vi "Actor Core.vi"(8 "error in":errorcluster, 11 "RandomDataChart in":refnum<class "AutoRegPanel.lvclass">) -> (0 "error out":errorcluster, 3 "Actor out":refnum<class "Actor.lvclass">)   [LabVIEW 2015, in "TestViewables.lvlib" / "AutoRegPanel.lvclass"]
doc: "(<B>Filename</B>: Actor Framework.lvlib:Actor.lvclass:Actor Core.vi)\n\nReceives messages to the actor, reacts to them, and initiates any error handling that may shut the actor down.\n\nDescendant classes may override this VI to append parallel tasks for the actor to complete while it handles messages. Overrides use the Call Parent Method node.\n\n<License>\nCopyright © 2017 Composed Systems, LLC | All rights reserved\nwww.composed.io\n\nAuthor: Ethan Stern <ethan.stern@composed.io>\n\nThis software is provided \"AS IS\" WITHOUT WARRANTIES, either express or implied, AND IS FOR EDUCATIONAL PURPOSES ONLY.\n</License>"
uses:
  AutoRegPanel.lvclass
  <vilib>/ActorFramework/Actor/Actor.lvclass
  <vilib>/ActorFramework/Actor/Actor.lvclass/Actor.ctl
  <vilib>/ActorFramework/Message Enqueuer/Message Enqueuer.lvclass/Message Enqueuer.ctl
  <vilib>/ActorFramework/Message Enqueuer/Init from Existing Queue.vi
  Framework/IViewable/IViewable/IViewable.lvclass
  <vilib>/ActorFramework/Message Enqueuer/Message Enqueuer.lvclass
  Framework/AutoRegistration/AutoRegistration/AutoRegistration.lvclass
  Framework/AutoRegistration/ActorAutoRegistration Messages/ValueChangeMsg/ValueChangeMsg.lvclass
panel:
  in  "Whitaker":bool caption="Latch When Released"
  in  "Walton":bool caption="Latch Until Released"
  in  "Launch Dialog":bool
  in  "Guthrie":bool caption="Switch Until Released"
  in  "Harrelson":bool caption="Switch When Released"
  in  "Gump":bool caption="Latch When Pressed"
  in  "Wilson":bool caption="Switch When Pressed"
  # "An actor implementing\ngeneral auto-reg in core"
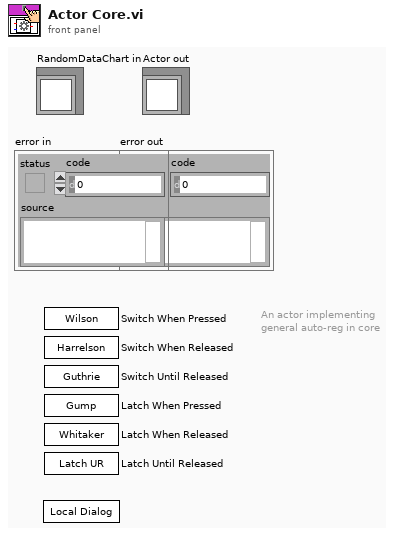
[diagram p1: front panel]
types:
  T1 = typedef "AutoRegistration.lvlib/AutoRegistration.lvclass/Auto-Event Registration Refnum.ctl" = refnum<event-registration>
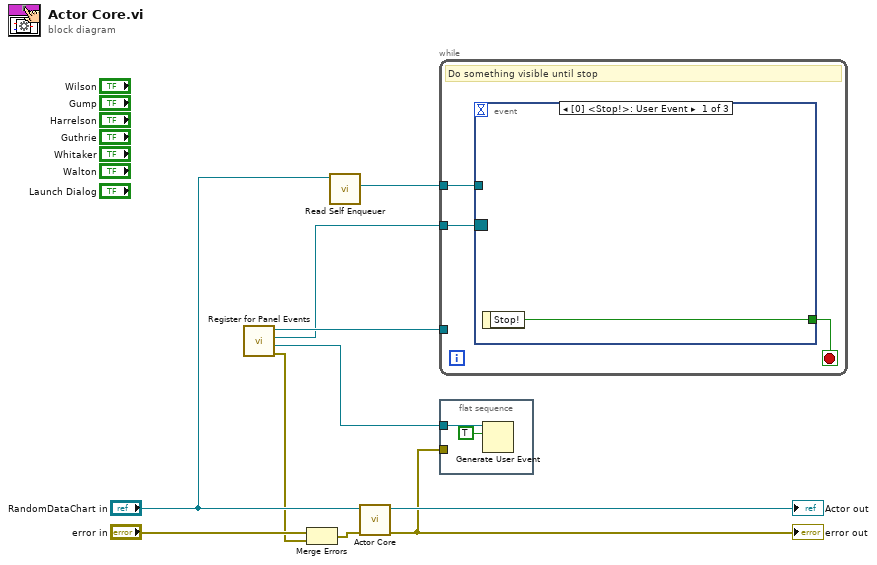
[diagram p0: block diagram]
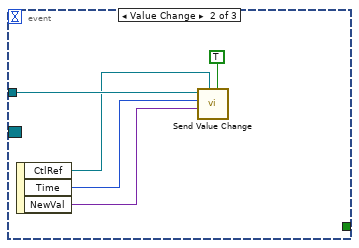
[diagram p2: hidden frame]
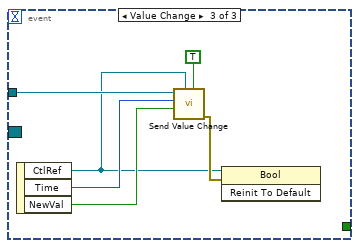
[diagram p3: hidden frame]
diagram:
  n1 = call "Register for Panel Events.vi"() -> ("error out"=w3:errorcluster, "Stop! Event"=w5:refnum<user-event>, "Auto-Event Registration Refnum"=w1:T1, "AbstractAutoRegistration out"=w2:refnum<class "AutoRegistration.lvclass">)  [unwired: 8 in]
  n2 = Merge Errors("error in", w3) -> (w4:errorcluster)
  n3 = call <vilib>:"Read Self Enqueuer.vi"("Actor"="RandomDataChart in") -> ("Self Enqueuer"=w6:refnum<class "Message Enqueuer.lvclass">)  [unwired: 10 in]
  n4 = call-parent "Actor Core.vi"("error in"=w4, "IViewable In"="RandomDataChart in") -> ("error out"=w8:errorcluster, "Actor out"=→"Actor out":refnum<class "Actor.lvclass">)  [unwired: 8 in]
  "error out" <- w8
  n5 = while {
    tunnel: w6 -> [w12]
    tunnel: w2 -> [_]
    tunnel: w1 -> [w11]
    stop <- w13 stop-if-true
    # "Do something visible until stop"
    n6 = event shown="[0] <Stop!>: User Event" {
      selector: w11 -> [_ _ _]
      dyn-events: _ -> [_ _ _]
      timeout: _ -> [_ _ _]
      tunnel: [w14 _ _] -> w13
      tunnel: w12 -> [_ w19 w25]
      event User Event {
        n7 = event-data() -> ("Stop!"=w14:bool)  [unwired: 1 in]
      }
      event Value Change {
        n8 = event-data() -> ("CtlRef"=w16:refnum<vi>, "Time"=w17:u32, "NewVal"=w18:variant)  [unwired: 1 in]
        n9 = call "Send Value Change.vi"("Use Label Text (F=Use Caption)"=TRUE, "Ctl Refnum"=w16, "New Value"=w18, "Time"=w17, "Message Enqueuer in"=w19) -> ()  [unwired: 6 in, 1 out]
      }
      event Value Change {
        n10 = event-data() -> ("CtlRef"=w21:refnum<vi>, "Time"=w23:u32, "NewVal"=w24:bool)  [unwired: 1 in]
        n11 = call "Send Value Change.vi"("Use Label Text (F=Use Caption)"=TRUE, "Ctl Refnum"=w21, "New Value"=w24, "Time"=w23, "Message Enqueuer in"=w25) -> ("error out"=w22:errorcluster)  [unwired: 6 in]
        n12 = invoke class="Bool" method="Reinit To Default"(reference=w21, error in=w22) -> ()  [unwired: 1 in, 3 out]
      }
    }
  }
  n13 = flat-sequence {
    tunnel: w5 -> [w27]
    tunnel: w8 -> [_]
    frame #0 {
      n14 = Generate User Event(user event=w27, event data cluster=TRUE ("event data")) -> ()  [unwired: 2 in, 2 out]
    }
  }
